vi "NXTLineLeader-Util-DM.vi"(0 "Input of NXTLineLeader-Util":T1={"Kp"=25, "Ki"=0, "Kd"=15, "SetPoint"=45, "Kp_factor"=32, "Ki_factor"=32, "Kd_factor"=32} {"Kd_factor" min=1; "Ki_factor" min=1; "Kp_factor" min=1; "SetPoint" max=80}, 2 "NXT":T3={"Hardware"="NXT", "Flattened String"=""}, 3 "Input Port":T2 items=["Port 1", "Port 2", "Port 3", "Port 4"]) -> (1 "Output of NXTLineLeader-Util":cluster{"Status":bool}, 4 "NXT dup":T3={"Hardware"="NXT", "Flattened String"=""} caption="NXT")   [LabVIEW 2010]
uses:
  <vilib>/NXT/Subs/LVHSConnector.ctl
  <vilib>/NXT/Block Support/NXT_InputPort.ctl
  <vilib>/NXT/Block Support/HWPage.SensorType.ctl
  <vilib>/NXT/Block Support/HWPage.SensorMode.ctl
panel:
  # "NXT_InputPort.ctlmindsensors.com\nCopyright (c) 2009 by mindsensors.com\nEmail: info (<at>) mindsensors (<dot>) com\n\nThis program is free software. You can redistribute it and/or modify\nit under the terms of the GNU General Public License as published by\nthe Free Software Foundation; version 3 of the License.\nRead the license at: http://www.gnu.org/licenses/gpl.txt"
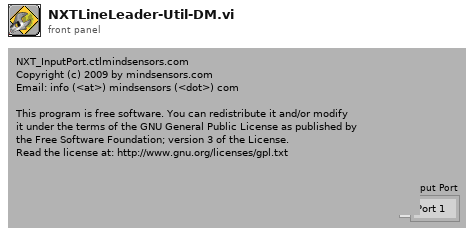
[diagram p1: front panel]
types:
  T1 = cluster{"Kp":u8, "Ki":u8, "Kd":u8, "SetPoint":u8, "Kp_factor":u8, "Ki_factor":u8, "Kd_factor":u8}
  T2 = typedef "NXT_InputPort.ctl" = u8
  T3 = typedef "LVHSConnector.ctl" = cluster{"Hardware":string, "Flattened String":string}
  T4 = typedef "HWPage.SensorType.ctl" = u8
  T5 = typedef "HWPage.SensorMode.ctl" = u8
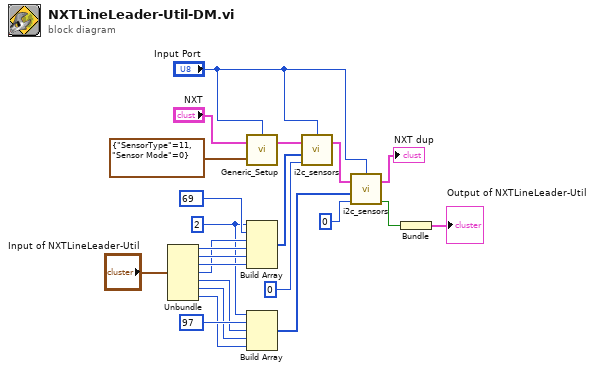
[diagram p0: block diagram]
diagram:
  w3 = u8 2 ("Select your \nDevice Address")
  n1 = Unbundle("Input of NXTLineLeader-Util") -> ("Kp"=w12:u8, "Ki"=w11:u8, "Kd"=w10:u8, "SetPoint"=w6:u8, "Kp_factor"=w9:u8, "Ki_factor"=w8:u8, "Kd_factor"=w7:u8)
  n2 = call <vilib>:"Generic_Setup.vi"("Sensor Setup"=cluster{"SensorType":T4, "Sensor Mode":T5} {"SensorType"=11, "Sensor Mode"=0}, "NXT"="NXT", "Port"="Input Port") -> ("NXT"=w20:T3)  [unwired: 1 out]
  n3 = Build Array(w3, u8 69 ("register"), w6, w12, w11, w10) -> (w18:u8[])
  n4 = Build Array(w3, i8 97 ("register"), w9, w8, w7) -> (w15:u8[])
  n5 = call <vilib>:"i2c_sensors.vi"("Return Length"=u8 0, "Bytes to Write"=w18, "NXT"=w20, "Port"="Input Port") -> ("NXT"=w21:T3)  [unwired: 1 in, 2 out]
  n6 = call <vilib>:"i2c_sensors.vi"("Return Length"=u8 0, "Bytes to Write"=w15, "NXT"=w21, "Port"="Input Port") -> ("Success?"=w2:bool, "NXT"=→"NXT dup":T3)  [unwired: 1 in, 1 out]
  n7 = Bundle("Success?"=w2) -> (→"Output of NXTLineLeader-Util":cluster{"Success?":bool})  [unwired: 1 in]
